vi "2-Byte Packed Mono to U16 2.vi"(0 "2-Byte Mono Data":u8[](array[numeric]) format="%08b", 1 "Image Size":T1, 2 "Bits":i32) -> (3 "U16 Pixels":u16[][](array[numeric]) format="%04x")   [LabVIEW 2020, in "Buffer.lvclass"]
uses:
  Image Size.ctl
  Buffer.lvclass
  Buffer.lvclass/Buffer.ctl
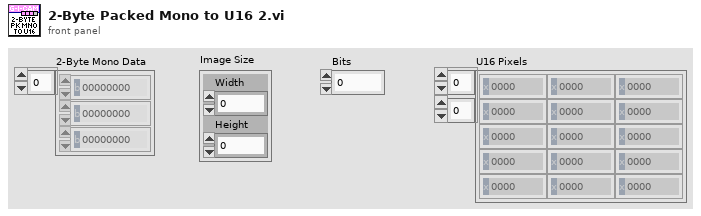
[diagram p1: front panel]
types:
  T1 = typedef "Buffer.lvclass/Image Size.ctl" = cluster{"Width":u16, "Height":u16}
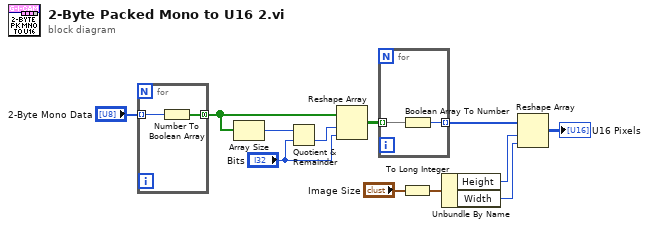
[diagram p0: block diagram]
diagram:
  n1 = for {
    tunnel: "2-Byte Mono Data" -> [w14] mode=indexing
    tunnel: [w13] -> w11 mode=concatenating
    n2 = Number To Boolean Array(number=w14) -> (Boolean array=w13:bool[])
  }
  n3 = Array Size(array=w11) -> (size(s)=w10:i32)
  n4 = Quotient & Remainder(x=w10, y="Bits") -> (floor(x/y)=w8:i32)  [unwired: 1 out]
  n5 = Reshape Array(w11, w8, "Bits") -> (w7:bool[][])
  n6 = for {
    tunnel: w7 -> [w16] mode=indexing
    tunnel: [w15] -> w6 mode=indexing
    n7 = Boolean Array To Number(Boolean array=w16) -> (number=w15:u16)
  }
  n8 = To Long Integer(number="Image Size") -> (32bit integer=w5:cluster{"Width":i32, "Height":i32})
  n9 = Unbundle By Name(w5) -> ("Height"=w4:i32, "Width"=w3:i32)
  n10 = Reshape Array(w6, w4, w3) -> (→"U16 Pixels":u16[][])
